vi "Check and Get Sizes.vi"(8 "error in (no error)":errorcluster, 9 "test commands":string[](array[string]), 10 "variable name":string, 11 "pipe in":T1) -> (0 "error out":errorcluster, 1 "octave sizes":i32[](array[numeric]), 2 "all tests OK?":bool, 3 "pipe out":T1)   [LabVIEW 2013, in "GOLPI library.lvlib"]
doc: "Checks GNU Octave variable and gets its size. 'variable name' is the name of the variable. 'test commands' is array of GNU Octave commands with boolean output applied to the variable. I.e. to read noncomplex double scalar variable 'x', following array should be supplied:\nisnumeric\nisscalar\n~isscomplex\nTests performed are:\nisnumeric(x)\nisscalar(x)\n~iscomplex(x)\nIf output of all tests is '1', output 'all tests OK?' is true.\nReturns size of variable in GNU Octave metric (i.e. no elements with zero indexes)"
uses:
  GOLPI library.lvlib
  LV Process.lvlibp/Pipe Handle.ctl
  Custom Error Codes Enum Type Def.vi
  Globals.vi
  LV Process.lvlibp
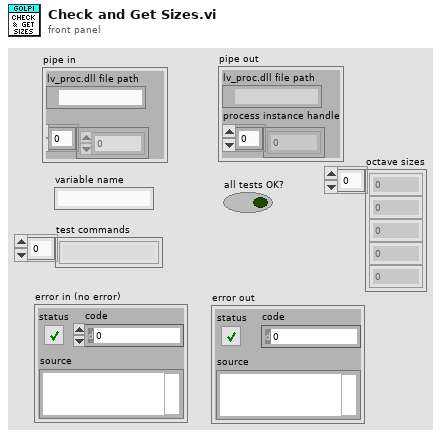
[diagram p1: front panel]
types:
  T1 = typedef "LV Process.lvlibp/Pipe Handle.ctl" = cluster{"lv_proc.dll file path":path, "process instance handle":u32[]}
  T2 = typedef "GOLPI library.lvlib/Custom Error Codes Enum Type Def.vi" = enum16{"no error", "00 working directory PAR1 missing", "01 octave binary PAR1 missing", "02 octave report error PAR1", "03 empty output last cmd PAR1", "04 missing temporary file PAR1", "10 var PAR1 not string", "11 var PAR1 not num, scal, ~compl", "12 var PAR1 not num, scal, compl", "13 var PAR1 not num, vect, ~compl", "14 var PAR1 not num, vect, compl", "15 var PAR1 not num, mat, ~compl", "16 var PAR1 not num, mat, ~compl", "99 not finished"}
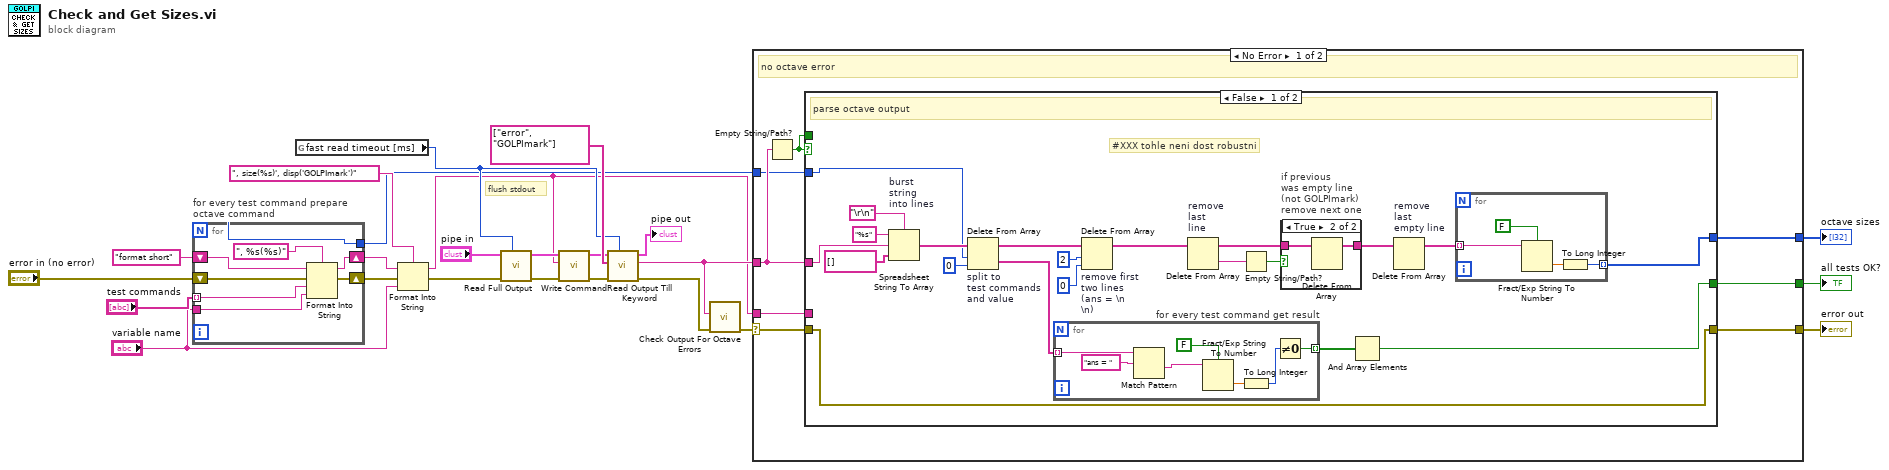
[diagram p0: block diagram]
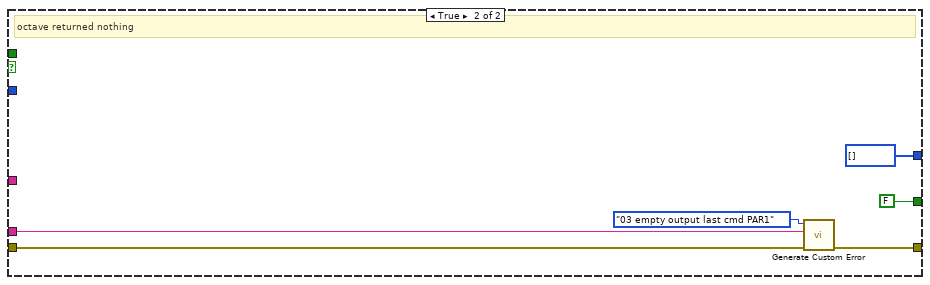
[diagram p3: hidden frame]
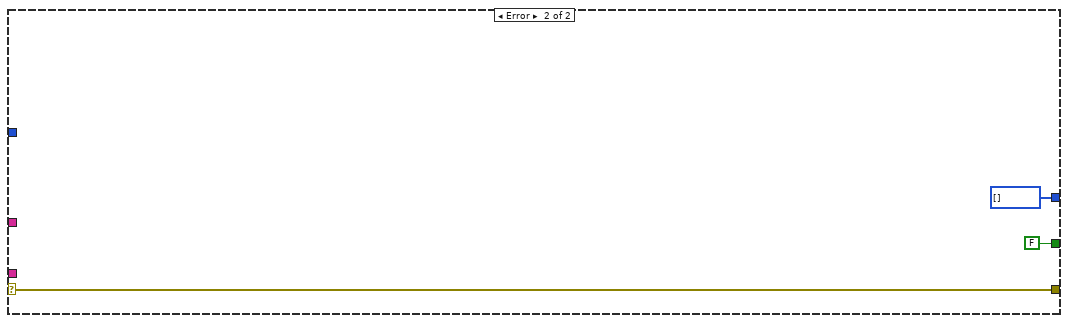
[diagram p4: hidden frame]
diagram:
  # "flush stdout"
  n1 = for "for every test command prepare\noctave command" {
    N -> [w25]
    tunnel: "test commands" -> [w30] mode=indexing
    tunnel: "variable name" -> [w29]
    shift-right: [w28] -> w18
    shift-left: "format short" -> [w31]
    shift-right: [w26] -> w19
    shift-left: "error in (no error)" -> [w27]
    tunnel: [w25] -> w1
    n2 = Format Into String(format string=", %s(%s)", initial string=w31, error in=w27, w30, w29) -> (resulting string=w28:string, error out=w26:errorcluster)
  }
  n3 = global read "Globals.vi" "fast read timeout [ms]"() -> (w10:u32)
  n4 = Format Into String(format string=", size(%s)', disp('GOLPImark')", initial string=w18, error in=w19, "variable name") -> (resulting string=w2:string, error out=w15:errorcluster)
  n5 = call "Read Full Output.vi"("timeout [ms]"=w10, "error in"=w15, "pipe in"="pipe in") -> ("error out"=w14:errorcluster, "pipe out"=w13:T1)  [unwired: 5 in, 2 out]
  n6 = call "Write Command.vi"("error in"=w14, "command"=w2, "pipe in"=w13) -> ("error out"=w8:errorcluster, "pipe out"=w9:T1)  [unwired: 7 in]
  n7 = call "Read Output Till Keyword.vi"("timeout [ms]"=w10, "error in"=w8, "keywords"=string[] ["error", "GOLPImark"], "pipe in"=w9) -> ("error out"=w6:errorcluster, "read buffer"=w5:string, "pipe out"=→"pipe out":T1)  [unwired: 4 in, 1 out]
  n8 = call "Check Output For Octave Errors.vi"("error in"=w6, "read buffer"=w5) -> ("error out"=w4:errorcluster)  [unwired: 9 in]
  n9 = case shown="No Error" w4 {
    selector: w4 -> [w37 w82]
    tunnel: [w40 FALSE] -> w20
    tunnel: [w39 i32[] []] -> w16
    tunnel: w5 -> [w38 _]
    tunnel: [w35 w82] -> w3
    tunnel: w2 -> [w34 _]
    tunnel: w1 -> [w33 _]
    frame No Error {
      # "no octave error"
      n10 = Empty String/Path?(string/path=w38) -> (empty?=w36:bool)
      n11 = case shown="False" w36 {
        tunnel: [w47 FALSE] -> w40
        tunnel: w36 -> [_ _]
        tunnel: [w41 i32[] []] -> w39
        tunnel: w38 -> [w52 _]
        tunnel: w37 -> [w51 w78]
        tunnel: [w51 w77] -> w35
        tunnel: w34 -> [_ w76]
        tunnel: w33 -> [w50 _]
        frame False {
          # "#XXX tohle neni dost robustni"
          # "parse octave output"
          n12 = Spreadsheet String To Array "burst\nstring\ninto lines"(delimiter (Tab)="\r\n", format string="%s", spreadsheet string=w52, array type (2D Dbl)=string[] []) -> (array=w58:string[])
          n13 = Delete From Array "split to\ntest commands\nand value"(array=w58, length=w50, index=0) -> (deleted portion=w49:string[], array with subset deleted=w46:string[])
          n14 = for "for every test command get result" {
            tunnel: w49 -> [w72] mode=indexing
            tunnel: [w66] -> w48 mode=indexing
            n15 = Match Pattern(string=w72, regular expression="ans = ") -> (after substring=w68:string)  [unwired: 1 in, 3 out]
            n16 = Fract/Exp String To Number(use system decimal point (T)=FALSE, string=w68) -> (number=w69:dbl)  [unwired: 2 in, 1 out]
            n17 = To Long Integer(number=w69) -> (32bit integer=w70:i32)
            n18 = Not Equal To 0?(x=w70) -> (x != 0?=w66:bool)
          }
          n19 = Delete From Array "remove first\ntwo lines\n(ans = \\n\n\\n)"(array=w46, length=2, index=0) -> (array with subset deleted=w43:string[])  [unwired: 1 out]
          n20 = Delete From Array "remove\nlast\nline"(array=w43) -> (deleted portion=w56:string, array with subset deleted=w55:string[])  [unwired: 2 in]
          n21 = Empty String/Path?(string/path=w56) -> (empty?=w53:bool)
          n22 = case "if previous\nwas empty line\n(not GOLPImark)\nremove next one" shown="True" w53 {
            tunnel: w55 -> [w73 w75]
            tunnel: [w73 w74] -> w54
            frame False {
            }
            frame True {
              n23 = Delete From Array(array=w75) -> (array with subset deleted=w74:string[])  [unwired: 2 in, 1 out]
            }
          }
          n24 = And Array Elements(Boolean array=w48) -> (logical AND=w47:bool)
          n25 = Delete From Array "remove\nlast\nempty line"(array=w54) -> (array with subset deleted=w42:string[])  [unwired: 2 in, 1 out]
          n26 = for {
            tunnel: w42 -> [w63] mode=indexing
            tunnel: [w62] -> w41 mode=indexing
            n27 = Fract/Exp String To Number(use system decimal point (T)=FALSE, string=w63) -> (number=w65:dbl)  [unwired: 2 in, 1 out]
            n28 = To Long Integer(number=w65) -> (32bit integer=w62:i32)
          }
        }
        frame True {
          # "octave returned nothing"
          n29 = call "Generate Custom Error.vi"("error in"=w78, "PAR1"=w76, "GOLPI error"=Custom_Error_Codes_Enum_Type_Def.vi."03 empty output last cmd PAR1" ("Enum")) -> ("error out"=w77:errorcluster)  [unwired: 8 in]
        }
      }
    }
    frame Error {
    }
  }
  "all tests OK?" <- w20
  "octave sizes" <- w16
  "error out" <- w3
